vi "Info Fix Indent.vi"(9 "Reduce multiple empty line (True)":bool=TRUE, 10 "indent string (8x space)":string="        ", 11 "info data in":string) -> (2 "lines":string[](array[string]), 3 "info data out":string)   [LabVIEW 2020]
doc: "Addition to infolib: Tries to fix line indentation to desired value. Note it may produce a mess when sections/matrices are corrupted. Also can remove multiple empty lines."
uses:
  <vilib>/regexp/Match Regular Expression.xnode
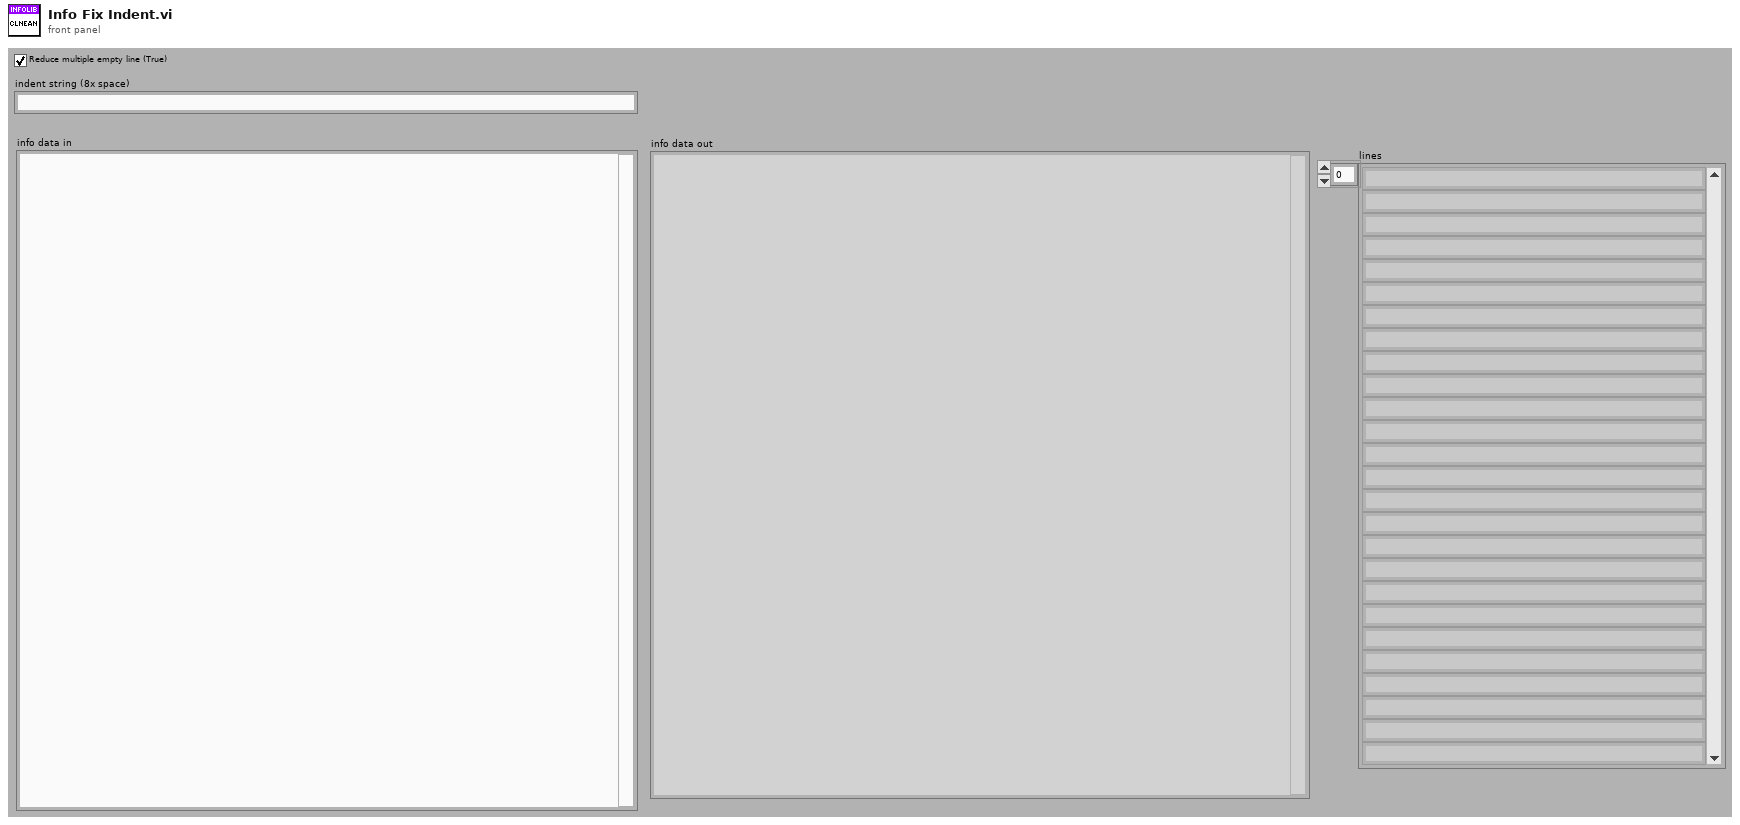
[diagram p1: front panel]
types:
  T1 = cluster{"submatch 2":string, "submatch 3":string}[]
  T2 = enum16{"Native", "Native Command Line", "UNIX", "Macintosh", "DOS"}
  T3 = cluster{"submatch 2":string, "submatch 3":string}
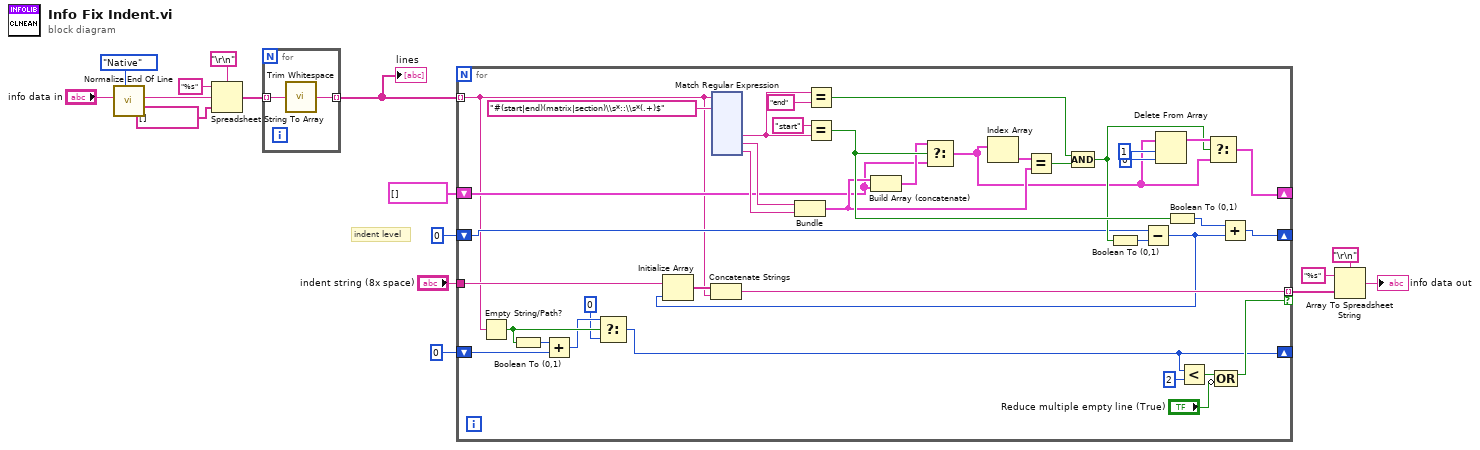
[diagram p0: block diagram]
diagram:
  # "indent level"
  n1 = call <vilib>:"Normalize End Of Line.vi"("end of line (Native)"=T2."Native", "string in"="info data in") -> ("string out"=w12:string)  [unwired: 6 in]
  n2 = Spreadsheet String To Array(delimiter (Tab)="\r\n", format string="%s", spreadsheet string=w12, array type (2D Dbl)=string[] []) -> (array=w10:string[])
  n3 = for {
    tunnel: w10 -> [w18] mode=indexing
    tunnel: [w17] -> w9 mode=indexing
    n4 = call <vilib>:"Trim Whitespace.vi"("string"=w18) -> ("trimmed string"=w17:string)  [unwired: 1 in]
  }
  "lines" <- w9
  n5 = for {
    tunnel: w9 -> [w29] mode=indexing
    shift-right: [w44] -> _
    shift-left: T1 [] -> [w34]
    shift-right: [w32] -> _
    shift-left: 0 -> [w31]
    tunnel: "indent string (8x space)" -> [w43]
    tunnel: [w41] -> w5 mode=indexing if=w22
    shift-right: [w20] -> _
    shift-left: 0 -> [w28]
    n6 = Empty String/Path?(string/path=w29) -> (empty?=w26:bool)
    n7 = Boolean To (0,1)(Boolean=w26) -> (0, 1=w27:i16)
    n8 = Add(x=w27, y=w28) -> (x+y=w25:i32)
    n9 = Select(t=w25, s=w26, f=0) -> (s? t:f=w20:i32)
    n10 = xnode "Match Regular Expression"("input string"=w29, "regular expression"="#(start|end)(matrix|section)\\s*::\\s*(.+)$") -> ("submatch 1"=w39:string, "submatch 2"=w40:string, "submatch 3"=w54:string)  [unwired: 4 in, 5 out]
    n11 = Bundle("submatch 2"=w40, "submatch 3"=w54) -> (w36:T3)  [unwired: 1 in]
    n12 = Equal?(x=w39, y="end") -> (x = y?=w49:bool)
    n13 = Equal?(x="start", y=w39) -> (x = y?=w52:bool)
    n14 = Build Array (concatenate)(w36, w34) -> (w35:T1)
    n15 = Select(t=w35, s=w52, f=w34) -> (s? t:f=w33:T1)
    n16 = Index Array(array=w33) -> (element=w50:T3)  [unwired: 1 in]
    n17 = Equal?(x=w50, y=w36) -> (x = y?=w37:bool)
    n18 = Compound Arithmetic op=AND(w49, w37) -> (w38:bool)
    n19 = Boolean To (0,1)(Boolean=w38) -> (0, 1=w48:i16)
    n20 = Subtract(x=w31, y=w48) -> (x-y=w30:i32)
    n21 = Initialize Array(w43, w30) -> (w42:string[])
    n22 = Concatenate Strings(w42, w29) -> (w41:string)
    n23 = Delete From Array(array=w33, length=1, index=0) -> (array with subset deleted=w45:T1)  [unwired: 1 out]
    n24 = Boolean To (0,1)(Boolean=w52) -> (0, 1=w53:i16)
    n25 = Less?(x=w20, y=2) -> (x < y?=w23:bool)
    n26 = Select(t=w45, s=w38, f=w33) -> (s? t:f=w44:T1)
    n27 = Compound Arithmetic op=OR(w23, invert "Reduce multiple empty line (True)") -> (w22:bool)
    n28 = Add(x=w53, y=w30) -> (x+y=w32:i32)
  }
  n29 = Array To Spreadsheet String(delimiter (Tab)="\r\n", array=w5, 3:"%s" ("format string")) -> (spreadsheet string=→"info data out":string)
